vi "ERRORSTOP.vi"(0 "Command OK/ERROR Monitor":string, 1 "connection ID in":refnum<k5>, 2 "Input Command":string, 3 "Received Command":string, 4 "Total Command In/Output":string) -> ()   [LabVIEW 2016]
uses:
  GrobaLimitVoltage.vi
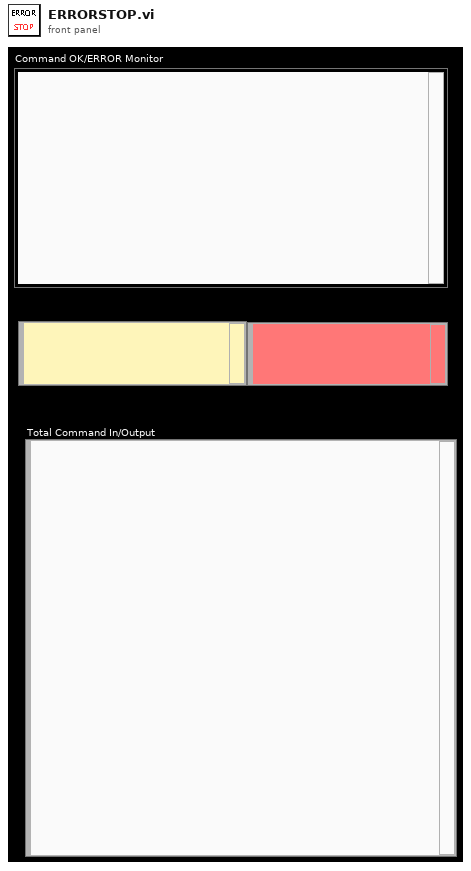
[diagram p1: front panel]
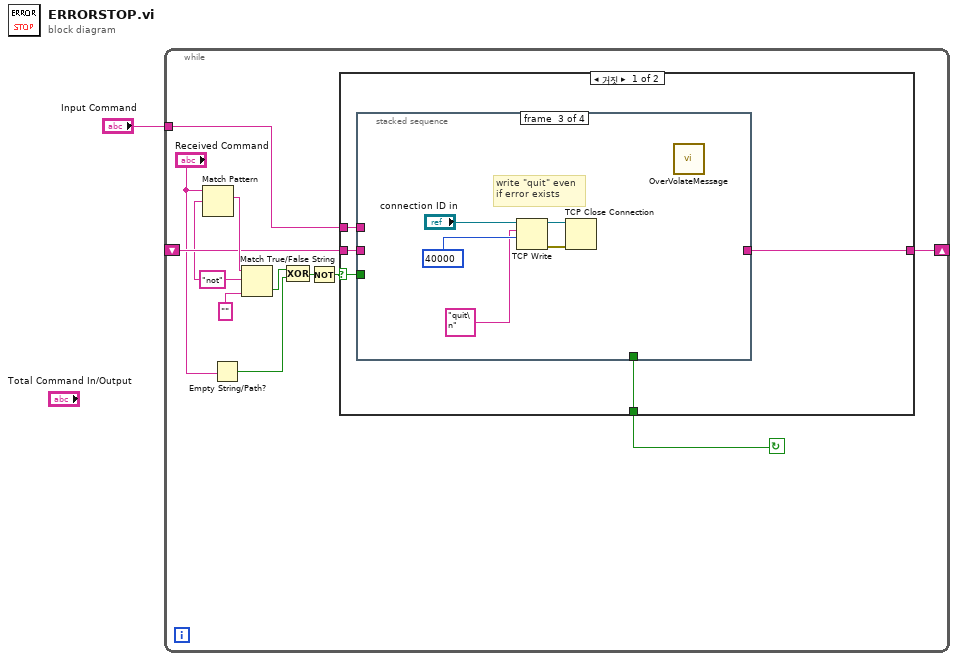
[diagram p0: block diagram]
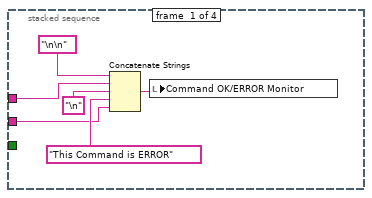
[diagram p2: hidden frame]
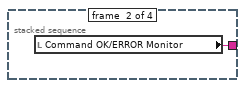
[diagram p3: hidden frame]
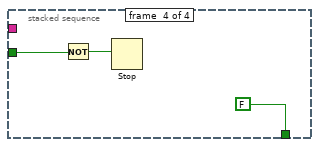
[diagram p4: hidden frame]
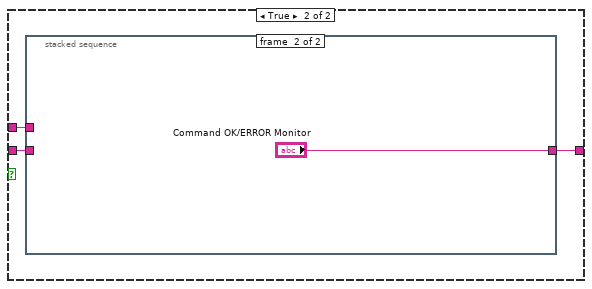
[diagram p5: hidden frame]
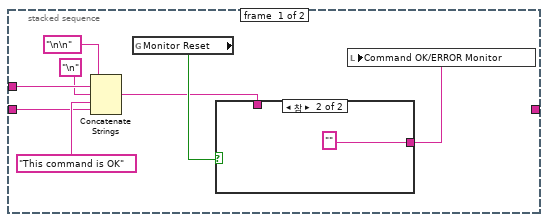
[diagram p6: hidden frame]
diagram:
  n1 = while {
    shift-right: [w12] -> _
    shift-left: _ -> [w11]
    tunnel: "Input Command" -> [w10]
    stop <- w9 continue-if-true
    w7 = "not" ("regular expression")
    n2 = Match Pattern(string="Received Command", regular expression=w7) -> (match substring=w13:string)  [unwired: 1 in, 3 out]
    n3 = Empty String/Path?(string/path="Received Command") -> (empty?=w2:bool)
    n4 = Match True/False String(2:"" ("true string"), 3:w7, 4:w13) -> (0:w5:bool)  [unwired: 1 out]
    n5 = Compound Arithmetic op=XOR(w5, w2) -> (w6:bool)
    n6 = Not(x=w6) -> (.not. x?=w4:bool)
    n7 = case shown="거짓" w4 {
      selector: w4 -> [w14 _]
      tunnel: w10 -> [w18 w36]
      tunnel: [w16 w34] -> w12
      tunnel: w11 -> [w17 w35]
      tunnel: [w15 _] -> w9
      frame False {
        n8 = stacked-sequence {
          tunnel: w18 -> [w24 _ _ _]
          tunnel: w17 -> [w19 _ _ _]
          tunnel: [_ w25 _ _] -> w16
          tunnel: [_ _ _ FALSE] -> w15
          tunnel: w14 -> [_ _ _ w32]
          frame #0 {
            n9 = Concatenate Strings("\n\n", w24, "\n", "This Command is ERROR" ("element"), w19) -> (w20:string)
            n10 = local write "Command OK/ERROR Monitor"(w20) -> ()
          }
          frame #1 {
            n11 = local read "Command OK/ERROR Monitor"() -> (w25:string)
          }
          frame #2 {
            # "write \"quit\" even\nif error exists"
            n12 = TCP Write(connection ID="connection ID in", data in="quit\n", 9:40000) -> (connection ID out=w30:refnum<k5>, error out=w29:errorcluster)  [unwired: 1 in, 1 out]
            n13 = TCP Close Connection(connection ID=w30, error in (no error)=w29) -> ()  [unwired: 1 in, 2 out]
            n14 = call "OverVolateMessage.vi"() -> ()  [unwired: 1 in]
          }
          frame #3 {
            n15 = Not(x=w32) -> (.not. x?=w33:bool)
            n16 = Stop(stop? (T)=w33) -> ()
          }
        }
      }
      frame True {
        n17 = stacked-sequence {
          tunnel: w36 -> [w44 _]
          tunnel: w35 -> [w40 _]
          tunnel: [_ "Command OK/ERROR Monitor"] -> w34
          frame #0 {
            n18 = Concatenate Strings("\n\n", w44, "\n", "This command is OK", w40) -> (w37:string)
            n19 = global read "GrobaLimitVoltage.vi" "Monitor Reset"() -> (w39:bool)
            n20 = case shown="참" w39 {
              tunnel: [w45 ""] -> w38
              tunnel: w37 -> [w45 _]
              frame False {
              }
              frame True {
              }
            }
            n21 = local write "Command OK/ERROR Monitor"(w38) -> ()
          }
          frame #1 {
          }
        }
      }
    }
  }
